vi "Save Protocol Settings.vi"() -> ()   [LabVIEW 2021]
panel:
  out "value":T1
  in  "JSON File Name":string
  in  "Bit Clock Edge  Sync":enum16{"Rising", "Falling"}(ring)=enum."Falling"
  in  "Frame Sync Pulse Width":i32=32
  in  "Frame Length":i32=64
  in  "Channel 0 Offset":i32=1
  in  "Bit Depth":i32=24
  in  "Channel Length":i32=32
  in  "Channel Count Per Frame":i32=2
  in  "Data Justification":enum16{"Left Justified", "Right Justified"}(ring)
  in  "Endianness":enum16{"MSB First", "LSB First"}(ring)
  in  "Frame Sync Edge for Channel 0":enum16{"Rising", "Falling"}(ring)
  out "JSON string":string
  # "Configurations"
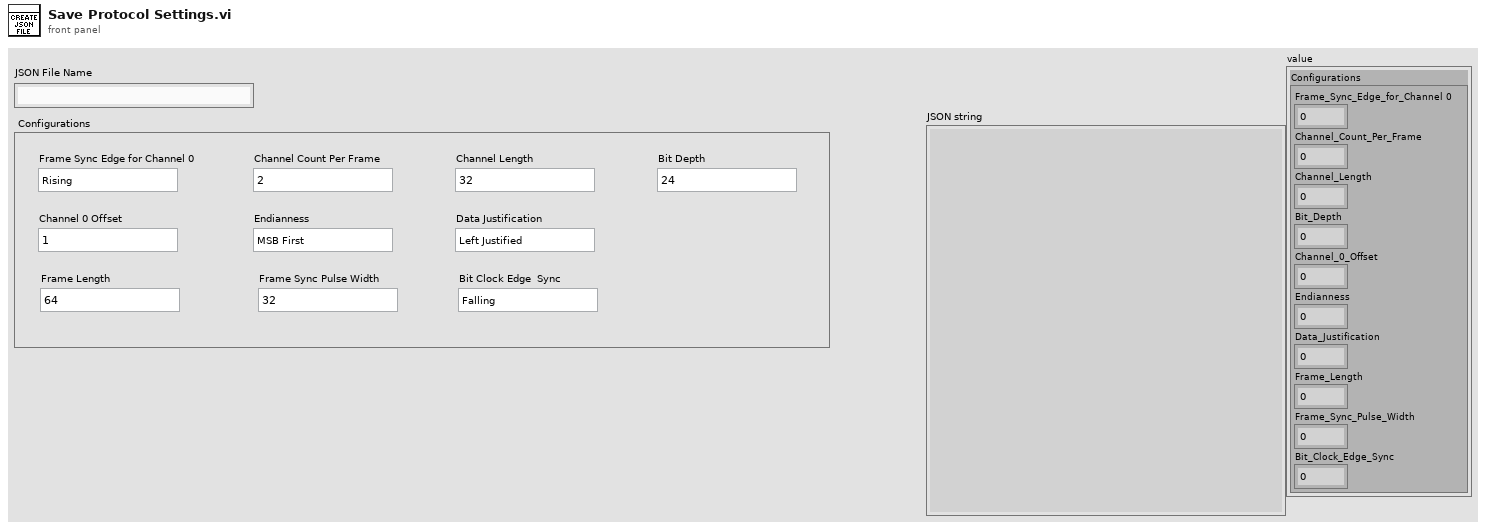
[diagram p1: front panel]
types:
  T1 = cluster{"Configurations":cluster{"Frame_Sync_Edge_for_Channel 0":i32, "Channel_Count_Per_Frame":i32, "Channel_Length":i32, "Bit_Depth":i32, "Channel_0_Offset":i32, "Endianness":i32, "Data_Justification":i32, "Frame_Length":i32, "Frame_Sync_Pulse_Width":i32, "Bit_Clock_Edge_Sync":i32}}
  T2 = enum16{"open", "replace", "create", "open or create", "replace or create", "replace or create with confirmation"}
  T3 = cluster{"Frame_Sync_Edge_for_Channel 0":i32, "Channel_Count_Per_Frame":i32, "Channel_Length":i32, "Bit_Depth":i32, "Channel_0_Offset":i32, "Endianness":i32, "Data_Justification":i32, "Frame_Length":i32, "Frame_Sync_Pulse_Width":i32, "Bit_Clock_Edge_Sync":i32}
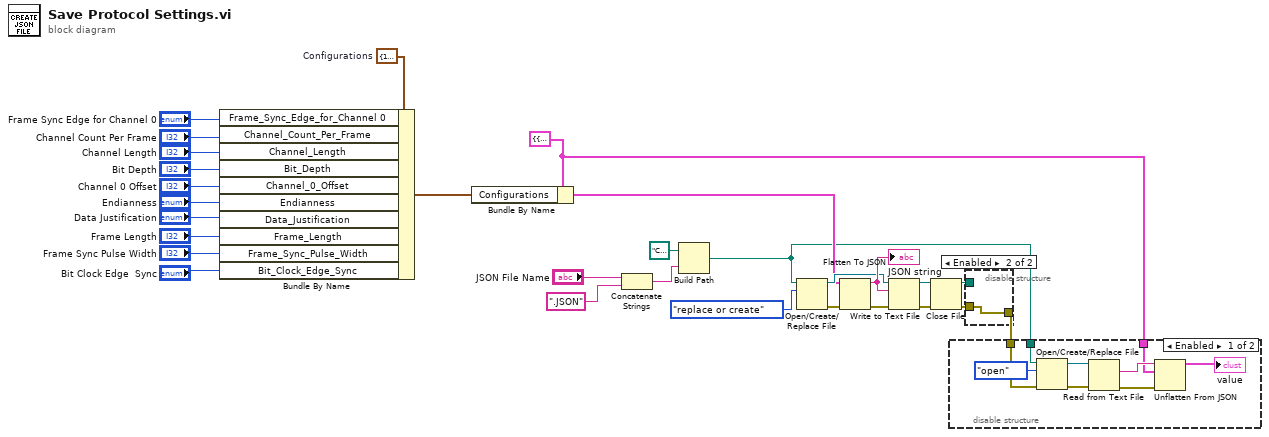
[diagram p0: block diagram]
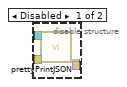
[diagram p2: hidden frame]
diagram:
  w1 = T1 {"Configurations"={"Frame_Sync_Edge_for_Channel 0"=1, "Channel_Count_Per_Frame"=2, "Channel_Length"=32, "Bit_Depth"=24, "Channel_0_Offset"=1, "Endianness"=0, "Data_Justification"=0, "Frame_Length"=0, "Frame_Sync_Pulse_Width"=0, "Bit_Clock_Edge_Sync"=0}}
  w29 = T3 {"Frame_Sync_Edge_for_Channel 0"=1, "Channel_Count_Per_Frame"=2, "Channel_Length"=32, "Bit_Depth"=24, "Channel_0_Offset"=1, "Endianness"=0, "Data_Justification"=0, "Frame_Length"=0, "Frame_Sync_Pulse_Width"=0, "Bit_Clock_Edge_Sync"=0}  # Configurations
  n1 = Bundle By Name(cluster=w29, "Frame_Sync_Edge_for_Channel 0"="Frame Sync Edge for Channel 0", "Channel_Count_Per_Frame"="Channel Count Per Frame", "Channel_Length"="Channel Length", "Bit_Depth"="Bit Depth", "Channel_0_Offset"="Channel 0 Offset", "Endianness"="Endianness", "Data_Justification"="Data Justification", "Frame_Length"="Frame Length", "Frame_Sync_Pulse_Width"="Frame Sync Pulse Width", "Bit_Clock_Edge_Sync"="Bit Clock Edge  Sync") -> (w5:T3)
  n2 = Bundle By Name(cluster=w1, "Configurations"=w5) -> (w19:T1)
  n3 = Concatenate Strings("JSON File Name", ".JSON" ("string")) -> (w7:string)
  n4 = Build Path(base path=path "C:/Users/Public/Documents/National Instruments/Audio/Protocols", name or relative path=w7) -> (appended path=w9:path)
  n5 = Open/Create/Replace File(file path (use dialog)=w9, operation (0:open)=T2."replace or create") -> (refnum out=w22:refnum<file>, error out=w20:errorcluster)  [unwired: 4 in, 1 out]
  n6 = Flatten To JSON(anything=w19, error in (no error)=w20) -> (JSON string=w26:string, 11:w25:errorcluster)  [unwired: 1 in]
  "JSON string" <- w26
  n7 = Write to Text File(file (use dialog)=w22, text=w26, error in=w25) -> (refnum out=w28:refnum<file>, error out=w24:errorcluster)  [unwired: 1 in, 1 out]
  n8 = Close File(refnum=w28, error in=w24) -> (path=w27:path, error out=w23:errorcluster)
  n9 = disable-structure shown="Enabled" {
    disable-tunnel: w27 -> [w32 _]
    disable-tunnel: w23 -> [w31 w33]
    disable-tunnel: [w30 w33] -> w18
    frame Disabled {
      n10 = call "prettyPrintJSON.vi"("error in"=w31, "JSON Path"=w32) -> ("error out"=w30:errorcluster)  [unwired: 7 in, 2 out]
    }
    frame Enabled {
    }
  }
  n11 = disable-structure shown="Enabled" {
    disable-tunnel: w18 -> [w42 _]
    disable-tunnel: w9 -> [w41 _]
    disable-tunnel: w1 -> [w35 _]
    frame Enabled {
      n12 = Open/Create/Replace File(file path (use dialog)=w41, error in=w42, operation (0:open)=T2."open") -> (refnum out=w37:refnum<file>, error out=w39:errorcluster)  [unwired: 3 in, 1 out]
      n13 = Read from Text File(file (use dialog)=w37, error in=w39) -> (text=w36:string, error out=w38:errorcluster)  [unwired: 2 in, 2 out]
      n14 = Unflatten From JSON(JSON string=w36, type and defaults=w35, error in (no error)=w38) -> (value=→"value":T1)  [unwired: 4 in, 1 out]
    }
    frame Disabled {
    }
  }
